vi "Scripting_ChangeNativeBaseClassInSubClass.vi"(0 "SubClass":refnum<vi>, 1 "NewBaseClass":path=path "C:/Projects/Base2_class/Base2.lvclass", 5 "error in (no error)":errorcluster) -> (19 "error out":errorcluster={"status"=TRUE, "code"=1055, "source"="Property Node in Scripting_ConvertBaseClassToSubClass.vi"})   [LabVIEW 2020]
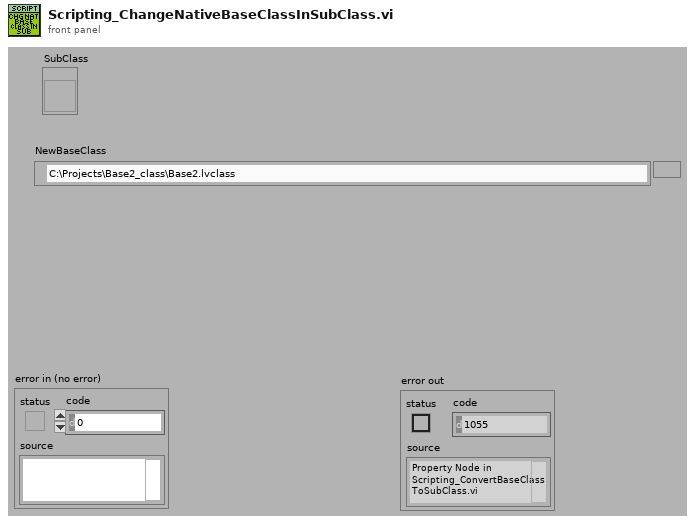
[diagram p1: front panel]
types:
  T1 = cluster{"NewBaseClass":refnum<vi>, "NewBaseClassPath":path, "SubClass":refnum<vi>, "NewBaseClassName":string, "AllBaseClassFiles":path[], "ClassVIs":refnum<vi>[], "CurrentBaseClassRef":refnum<vi>, "CurrentBaseClassPath":path, "CurrentRootBaseClassPath":path, "NewRootBaseClassPath":path, "ProtectedAttrbuts":bool, "ChangeToBase":bool, "App":refnum<vi>}
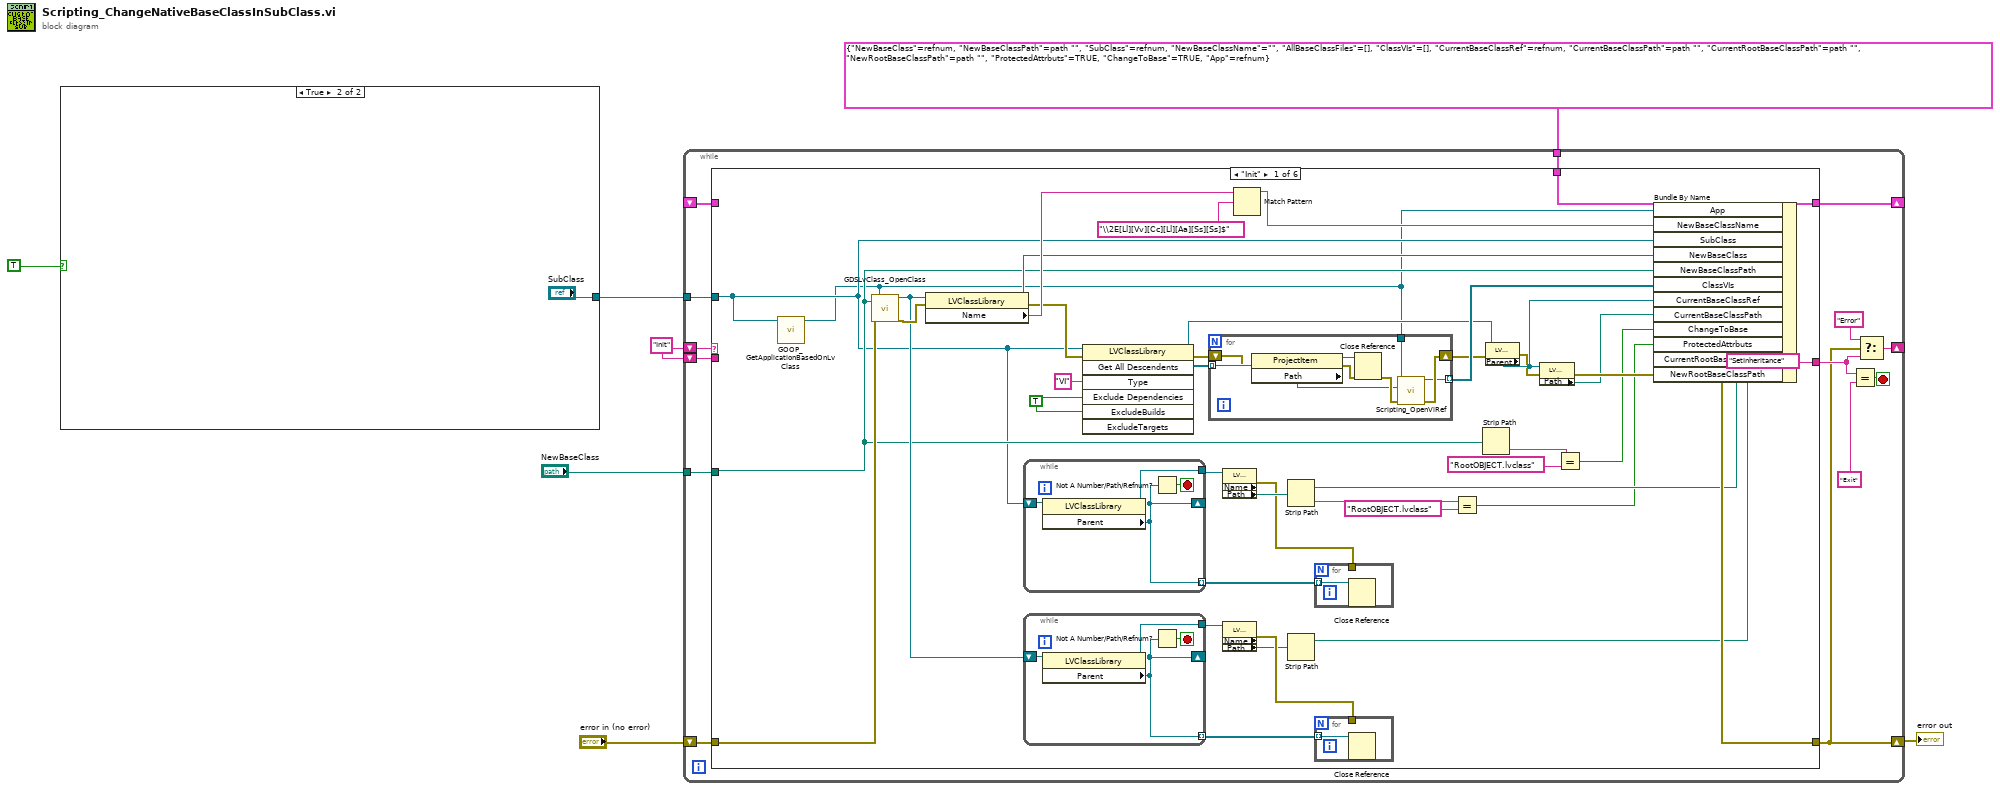
[diagram p0: block diagram]
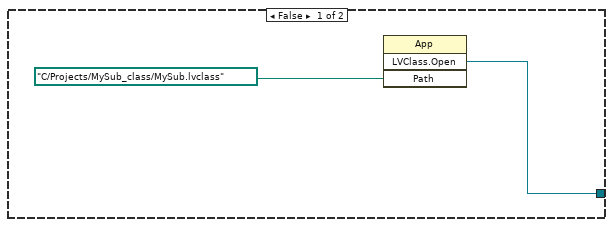
[diagram p2: hidden frame]
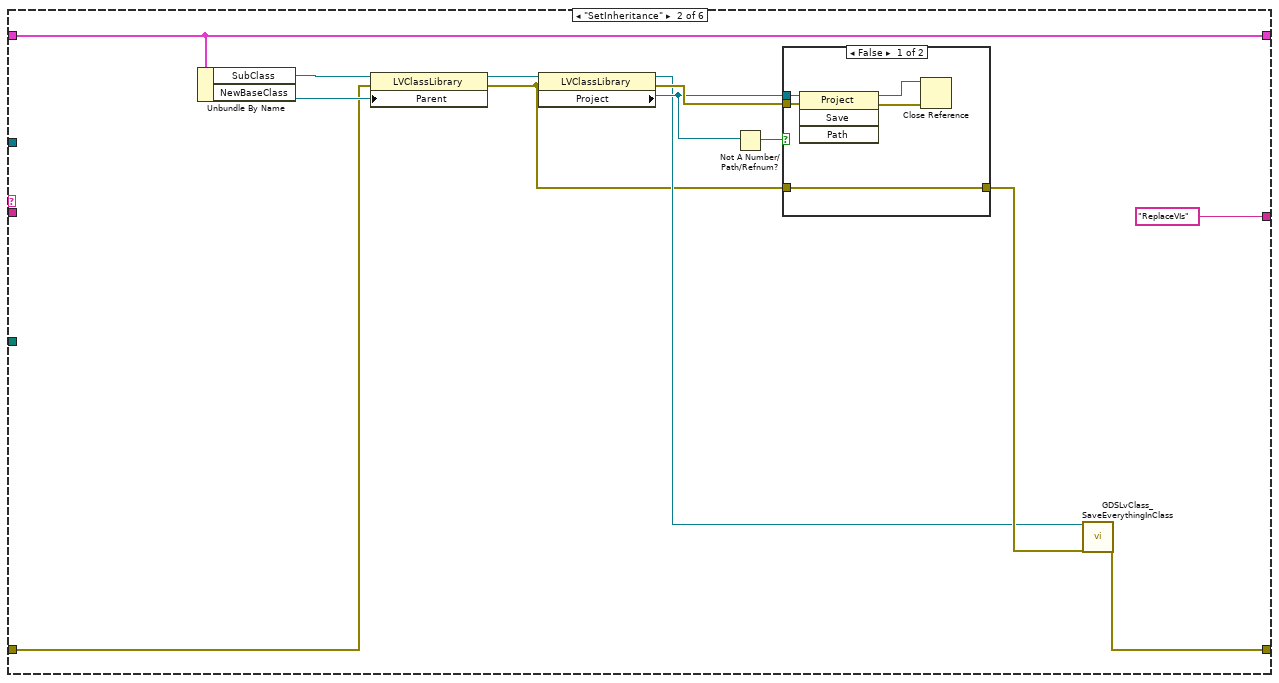
[diagram p3: hidden frame]
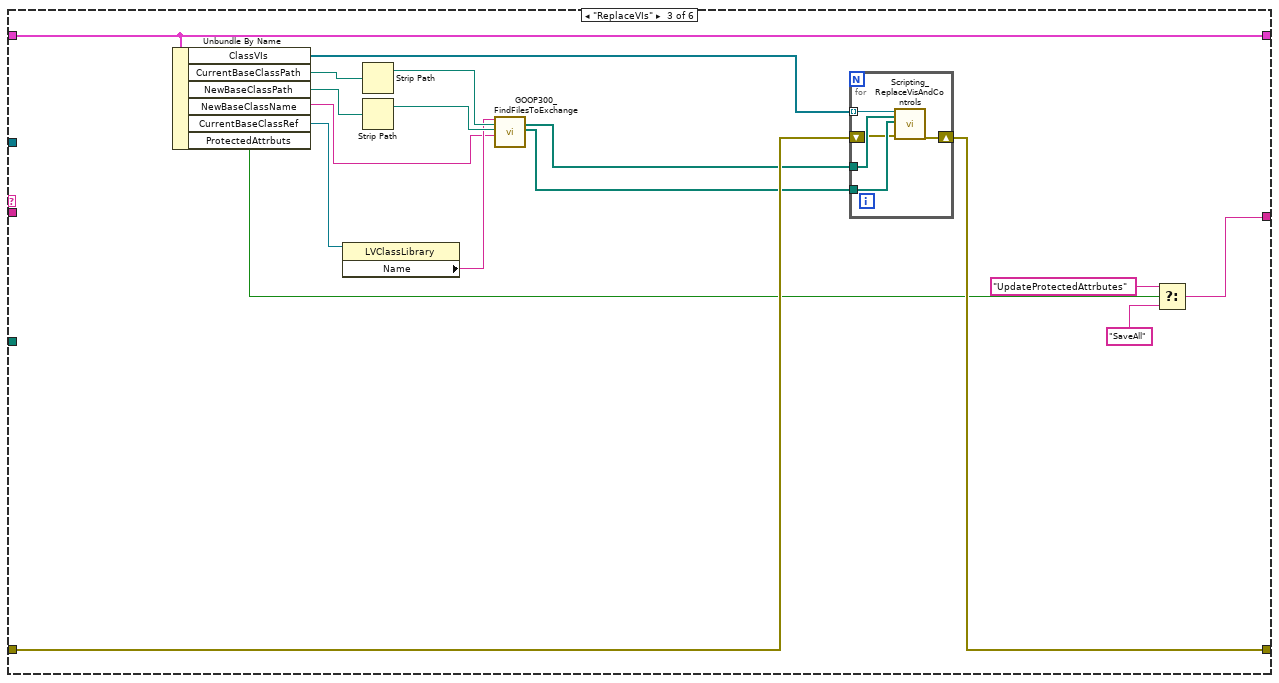
[diagram p5: hidden frame]
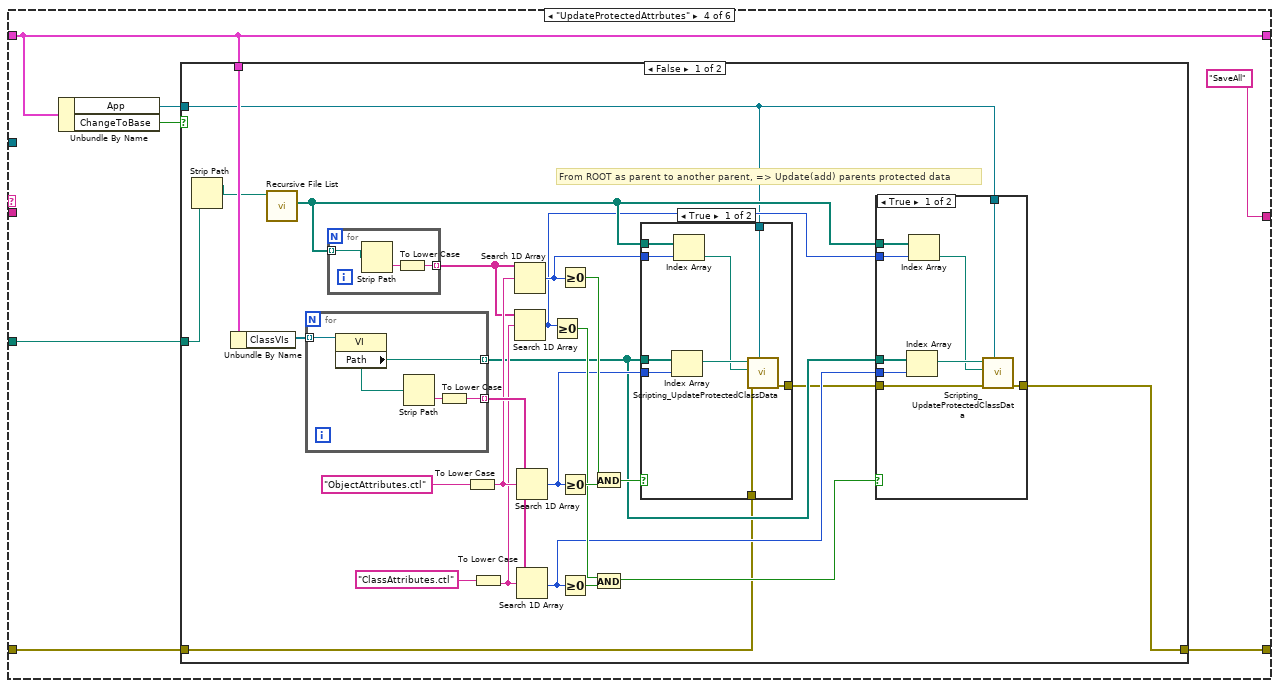
[diagram p6: hidden frame]
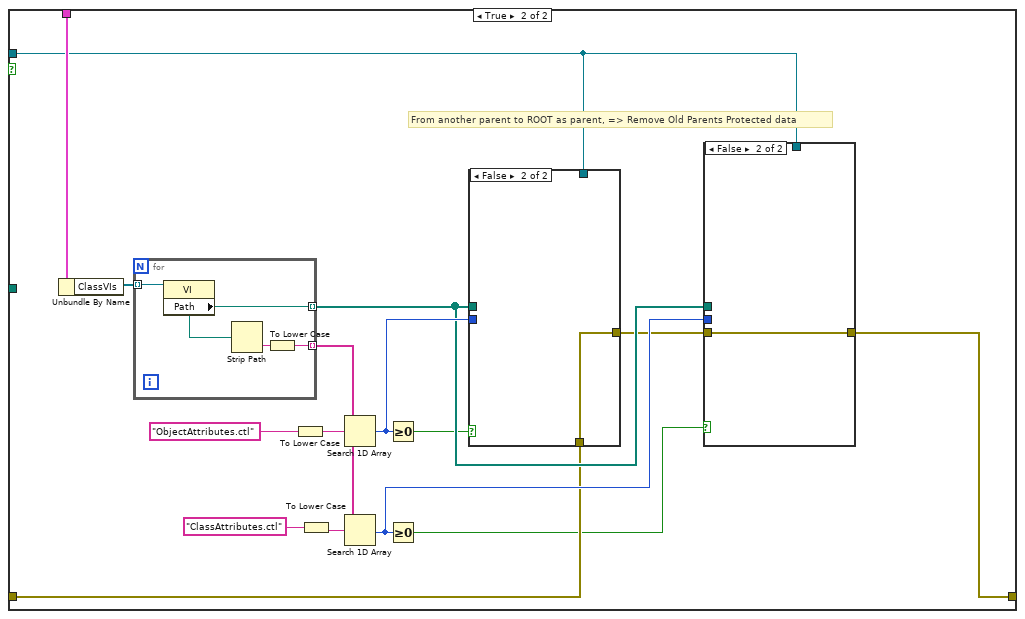
[diagram p9: hidden frame]
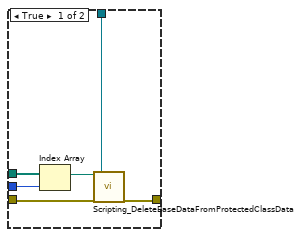
[diagram p10: hidden frame]
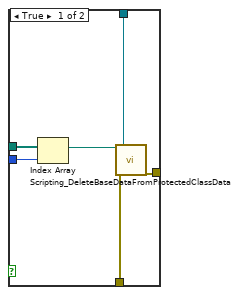
[diagram p11: hidden frame]
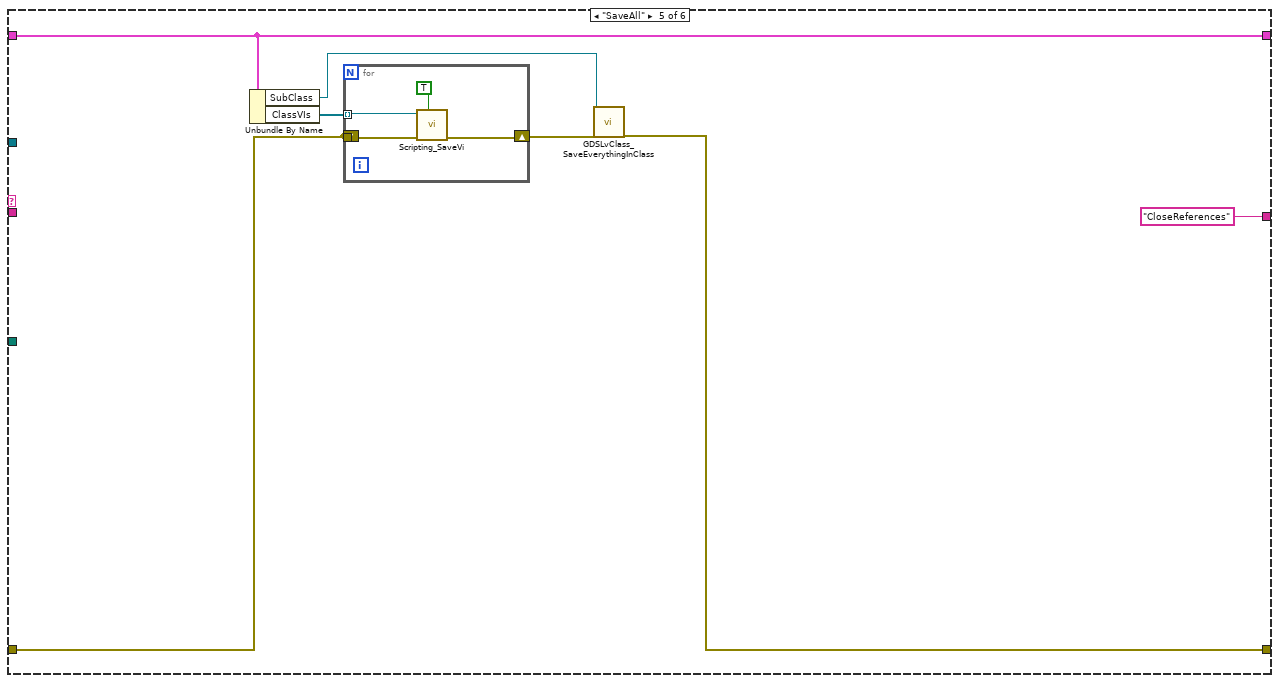
[diagram p12: hidden frame]
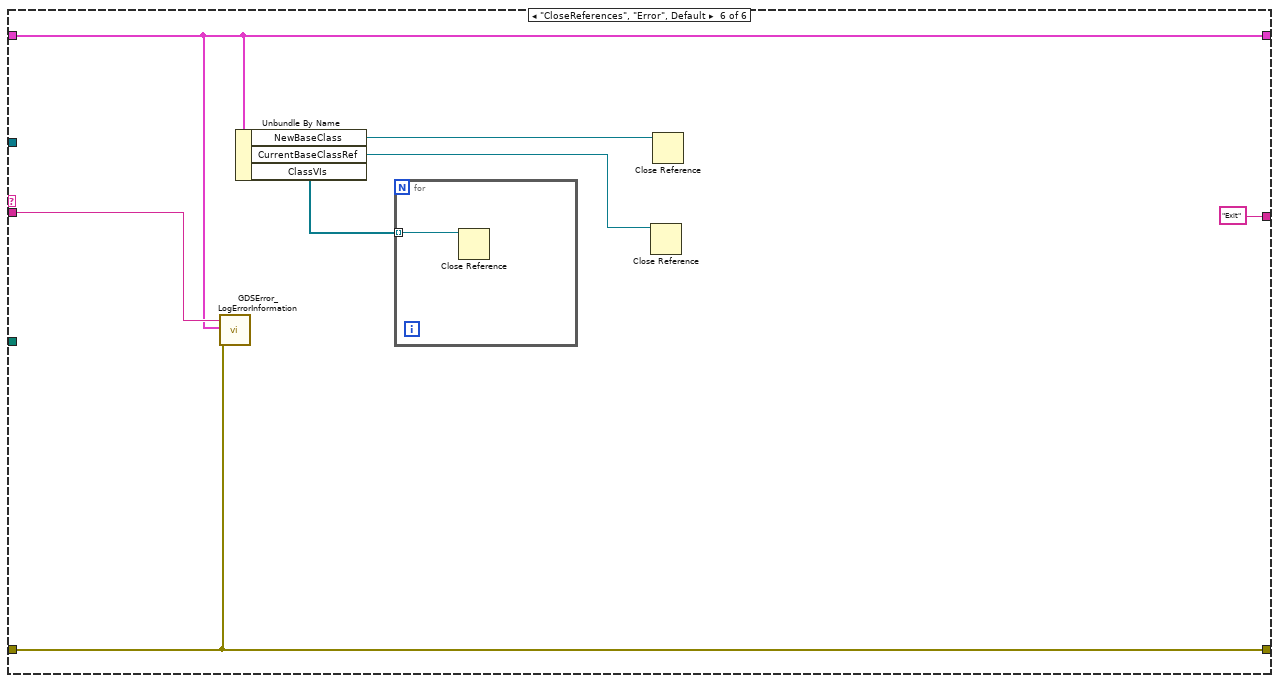
[diagram p13: hidden frame]
diagram:
  w1 = "Init"
  n1 = case shown="True" TRUE {
    tunnel: [w8 "SubClass"] -> w3
    frame False {
      n2 = invoke class="App" method="LVClass.Open"("Path"=path "C:/Projects/MySub_class/MySub.lvclass" ("vi path")) -> ("LVClass.Open"=w8:refnum<vi>)  [unwired: 3 in, 3 out]
    }
    frame True {
    }
  }
  n3 = while {
    shift-right: [w17] -> w6
    shift-left: "error in (no error)" -> [w24]
    shift-right: [w22] -> _
    shift-left: w1 -> [w23]
    shift-right: [w16] -> _
    shift-left: _ -> [w15]
    tunnel: w3 -> [w14]
    tunnel: T1 {"NewBaseClass"=refnum, "NewBaseClassPath"=path "", "SubClass"=refnum, "NewBaseClassName"="", "AllBaseClassFiles"=[], "ClassVIs"=[], "CurrentBaseClassRef"=refnum, "CurrentBaseClassPath"=path "", "CurrentRootBaseClassPath"=path "", "NewRootBaseClassPath"=path "", "ProtectedAttrbuts"=TRUE, "ChangeToBase"=TRUE, "App"=refnum} -> [w13]
    tunnel: "NewBaseClass" -> [w12]
    shift-left: w1 -> [w11]
    stop <- w21 stop-if-true
    n4 = case shown="\"Init\"" w23 {
      tunnel: w24 -> [w48 w94 w114 w132 w224 w233]
      tunnel: [w55 w85 w108 w129 w221 w233] -> w17
      tunnel: ["SetInheritance" "ReplaceVIs" w106 "SaveAll" "CloseReferences" "Exit"] -> w18
      tunnel: [w65 w96 w118 w128 w225 w231] -> w16
      tunnel: w15 -> [_ w96 w118 w128 w225 w231]
      tunnel: w14 -> [w26 _ _ _ _ _]
      tunnel: w13 -> [w62 _ _ _ _ _]
      tunnel: w12 -> [w31 _ _ w131 _ _]
      tunnel: w11 -> [_ _ _ _ _ w232]
      frame "Init" {
        w34 = TRUE ("ExcludeDependencies")
        n5 = call <resource>:"GOOP_GetApplicationBasedOnLvClass.vi"("LVClassLibrary in"=w26) -> ("Application out"=w25:refnum<vi>)  [unwired: 9 in, 1 out]
        n6 = call <resource>:"GDSLvClass_OpenClass.vi"("ClassToOpen"=w31, "error in (no error)"=w48, "Project/ApplicationRef(If empty, currect active project will be used)"=w25) -> ("LVClass.Open"=w36:refnum<vi>, "error out"=w49:errorcluster)  [unwired: 15 in]
        n7 = property class="LVClassLibrary"(reference=w36, error in=w49) -> (reference out=w46:refnum<vi>, error out=w47:errorcluster, "Name"=w60:string)
        n8 = while {
          shift-right: [w73] -> _
          shift-left: w26 -> [w74]
          tunnel: [w73] -> w45 mode=indexing
          tunnel: [w72] -> w44
          stop <- w75 stop-if-true
          n9 = property class="LVClassLibrary"(reference=w74) -> (reference out=w72:refnum<vi>, "Parent"=w73:refnum<vi>)  [unwired: 1 in, 1 out]
          n10 = Not A Number/Path/Refnum?(number/path/refnum=w73) -> (NaN/Path/Refnum?=w75:bool)
        }
        n11 = while {
          shift-right: [w68] -> _
          shift-left: w36 -> [w69]
          tunnel: [w68] -> w37 mode=indexing
          tunnel: [w67] -> w38
          stop <- w70 stop-if-true
          n12 = property class="LVClassLibrary"(reference=w69) -> (reference out=w67:refnum<vi>, "Parent"=w68:refnum<vi>)  [unwired: 1 in, 1 out]
          n13 = Not A Number/Path/Refnum?(number/path/refnum=w68) -> (NaN/Path/Refnum?=w70:bool)
        }
        n14 = invoke class="LVClassLibrary" method="Get All Descendents"(reference=w26, error in=w47, "Type"="VI", "Exclude Dependencies"=w34, "ExcludeBuilds"=w34) -> (reference out=w52:refnum<vi>, error out=w63:errorcluster, "All Descendents"=w64:refnum<vi>[])  [unwired: 2 in, 4 out]
        n15 = for {
          tunnel: w64 -> [w84] mode=indexing
          shift-right: [w79] -> w56
          shift-left: w63 -> [w81]
          tunnel: [w77] -> w57 mode=indexing
          tunnel: w25 -> [w76]
          n16 = property class="ProjectItem"(reference=w84, error in=w81) -> (reference out=w83:refnum<vi>, error out=w82:errorcluster, "Path"=w78:path)
          n17 = Close Reference(reference=w83, error in (no error)=w82) -> (error out=w80:errorcluster)
          n18 = call <resource>:"Scripting_OpenViRef.vi"("error in"=w80, "ViPath/ViName/Viref"=w78, "AppRef"=w76) -> ("error out"=w79:errorcluster, "vi reference"=w77:refnum<vi>)  [unwired: 6 in, 1 out]
        }
        n19 = property class="LVClassLibrary" props=["Name", "Path"](reference=w44) -> (error out=w42:errorcluster, "Path"=w43:path)  [unwired: 1 in, 2 out]
        n20 = property class="LVClassLibrary" props=["Name", "Path"](reference=w38) -> (error out=w40:errorcluster, "Path"=w39:path)  [unwired: 1 in, 2 out]
        n21 = Match Pattern(string=w60, regular expression="\\2E[Ll][Vv][Cc][Ll][Aa][Ss][Ss]$") -> (before substring=w59:string)  [unwired: 1 in, 3 out]
        n22 = Strip Path(path=w43) -> (stripped path=w41:path, name=w33:string)
        n23 = Strip Path(path=w39) -> (stripped path=w35:path)  [unwired: 1 out]
        n24 = for {
          tunnel: w45 -> [w71] mode=indexing
          tunnel: w42 -> [_]
          n25 = Close Reference(reference=w71) -> ()  [unwired: 1 in, 1 out]
        }
        n26 = for {
          tunnel: w37 -> [w66] mode=indexing
          tunnel: w40 -> [_]
          n27 = Close Reference(reference=w66) -> ()  [unwired: 1 in, 1 out]
        }
        n28 = Equal?(x=w33, y="RootOBJECT.lvclass") -> (x = y?=w27:bool)
        n29 = Strip Path(path=w31) -> (name=w30:string)  [unwired: 1 out]
        n30 = property class="LVClassLibrary"(reference=w52, error in=w56) -> (error out=w51:errorcluster, "Parent"=w54:refnum<vi>)  [unwired: 1 out]
        n31 = property class="LVClassLibrary"(reference=w54, error in=w51) -> (error out=w55:errorcluster, "Path"=w53:path)  [unwired: 1 out]
        n32 = Equal?(x=w30, y="RootOBJECT.lvclass") -> (x = y?=w28:bool)
        n33 = Bundle By Name(cluster=w62, "App"=w25, "NewBaseClassName"=w59, "SubClass"=w26, "NewBaseClass"=w46, "NewBaseClassPath"=w31, "ClassVIs"=w57, "CurrentBaseClassRef"=w54, "CurrentBaseClassPath"=w53, "ChangeToBase"=w28, "ProtectedAttrbuts"=w27, "CurrentRootBaseClassPath"=w41, "NewRootBaseClassPath"=w35) -> (w65:T1)
      }
      frame "SetInheritance" {
        n34 = Unbundle By Name(w96) -> ("SubClass"=w97:refnum<vi>, "NewBaseClass"=w95:refnum<vi>)
        n35 = property class="LVClassLibrary"(reference=w97, error in=w94, "Parent"=w95) -> (reference out=w92:refnum<vi>, error out=w86:errorcluster)
        n36 = property class="LVClassLibrary"(reference=w92, error in=w86) -> (reference out=w87:refnum<vi>, error out=w91:errorcluster, "Project"=w90:refnum<vi>)
        n37 = Not A Number/Path/Refnum?(number/path/refnum=w90) -> (NaN/Path/Refnum?=w89:bool)
        n38 = case shown="False" w89 {
          tunnel: w91 -> [w100 _]
          tunnel: w90 -> [w99 _]
          tunnel: w86 -> [w98 w103]
          tunnel: [w98 w103] -> w88
          frame False {
            n39 = invoke class="Project" method="Save"(reference=w99, error in=w100) -> (reference out=w101:refnum<vi>, error out=w102:errorcluster)  [unwired: 2 in, 2 out]
            n40 = Close Reference(reference=w101, error in (no error)=w102) -> ()  [unwired: 1 out]
          }
          frame True {
          }
        }
        n41 = call <resource>:"GDSLvClass_SaveEverythingInClass.vi"("ClassRefIn"=w87, "error in"=w88) -> ("error out"=w85:errorcluster)  [unwired: 16 in, 1 out]
      }
      frame "ReplaceVIs" {
        n42 = Unbundle By Name(w118) -> ("ClassVIs"=w117:refnum<vi>[], "CurrentBaseClassPath"=w120:path, "NewBaseClassPath"=w119:path, "NewBaseClassName"=w109:string, "CurrentBaseClassRef"=w111:refnum<vi>, "ProtectedAttrbuts"=w107:bool)
        n43 = property class="LVClassLibrary"(reference=w111) -> ("Name"=w110:string)  [unwired: 1 in, 2 out]
        n44 = Strip Path(path=w120) -> (stripped path=w116:path)  [unwired: 1 out]
        n45 = Strip Path(path=w119) -> (stripped path=w115:path)  [unwired: 1 out]
        n46 = call <resource>:"GOOP300_FindFilesToExchange.vi"("OldClassName(Prefix or suffix for some VIs)"=w110, "OldFolderPath"=w116, "NewFolderPath"=w115, "NewClassName(Prefix or suffix for some VIs)"=w109) -> ("OldFiles"=w113:path[], "NewFileArray"=w112:path[])  [unwired: 14 in]
        n47 = for {
          shift-right: [w125] -> w108
          shift-left: w114 -> [w122]
          tunnel: w113 -> [w124]
          tunnel: w112 -> [w123]
          tunnel: w117 -> [w121] mode=indexing
          n48 = call <resource>:"Scripting_ReplaceVisAndControls.vi"("ViRef"=w121, "OldVIsAndControls"=w124, "NewVIsAndControls"=w123, "error in (no error)"=w122) -> ("error out"=w125:errorcluster)  [unwired: 14 in, 1 out]
        }
        n49 = Select(t="UpdateProtectedAttrbutes", s=w107, f="SaveAll") -> (s? t:f=w106:string)
      }
      frame "UpdateProtectedAttrbutes" {
        n50 = Unbundle By Name(w128) -> ("App"=w126:refnum<vi>, "ChangeToBase"=w130:bool)
        n51 = case shown="False" w130 {
          tunnel: w132 -> [w138 w191]
          tunnel: w128 -> [w137 w190]
          tunnel: w131 -> [w135 _]
          tunnel: [w134 w189] -> w129
          tunnel: w126 -> [w133 w186]
          frame False {
            # "From ROOT as parent to another parent, => Update(add) parents protected data"
            n52 = Strip Path(path=w135) -> (stripped path=w136:path)  [unwired: 1 out]
            n53 = Unbundle By Name(w137) -> ("ClassVIs"=w158:refnum<vi>[])
            n54 = call <vilib>:"Recursive File List.vi"("Folder Path"=w136) -> ("All Files in Dir"=w144:path[])  [unwired: 6 in, 4 out]
            n55 = for {
              tunnel: w158 -> [w185] mode=indexing
              tunnel: [w184] -> w141 mode=indexing
              tunnel: [w182] -> w156 mode=indexing
              n56 = property class="VI"(reference=w185) -> ("Path"=w184:path)  [unwired: 1 in, 2 out]
              n57 = Strip Path(path=w184) -> (name=w183:string)  [unwired: 1 out]
              n58 = To Lower Case(string=w183) -> (all lower case string=w182:string)
            }
            n59 = for {
              tunnel: w144 -> [w170] mode=indexing
              tunnel: [w169] -> w150 mode=indexing
              n60 = Strip Path(path=w170) -> (name=w171:string)  [unwired: 1 out]
              n61 = To Lower Case(string=w171) -> (all lower case string=w169:string)
            }
            n62 = To Lower Case(string="ObjectAttributes.ctl") -> (all lower case string=w154:string)
            n63 = To Lower Case(string="ClassAttributes.ctl") -> (all lower case string=w149:string)
            n64 = Search 1D Array(1D array=w150, element=w154) -> (index of element=w145:i32)  [unwired: 1 in]
            n65 = Search 1D Array(1D array=w150, element=w149) -> (index of element=w143:i32)  [unwired: 1 in]
            n66 = Search 1D Array(1D array=w156, element=w154) -> (index of element=w146:i32)  [unwired: 1 in]
            n67 = Search 1D Array(1D array=w156, element=w149) -> (index of element=w140:i32)  [unwired: 1 in]
            n68 = Greater Or Equal To 0?(x=w143) -> (x >= 0?=w148:bool)
            n69 = Greater Or Equal To 0?(x=w145) -> (x >= 0?=w152:bool)
            n70 = Greater Or Equal To 0?(x=w146) -> (x >= 0?=w153:bool)
            n71 = Greater Or Equal To 0?(x=w140) -> (x >= 0?=w147:bool)
            n72 = And(x=w152, y=w153) -> (x .and. y?=w151:bool)
            n73 = And(x=w148, y=w147) -> (x .and. y?=w142:bool)
            n74 = case shown="True" w151 {
              tunnel: w138 -> [w180 w181]
              tunnel: w141 -> [w179 _]
              tunnel: w144 -> [w177 _]
              tunnel: w146 -> [w175 _]
              tunnel: w145 -> [w174 _]
              tunnel: [w173 w181] -> w139
              tunnel: w133 -> [w172 _]
              frame True {
                n75 = Index Array(array=w179, index=w175) -> (element=w178:path)
                n76 = Index Array(array=w177, index=w174) -> (element=w176:path)
                n77 = call <resource>:"Scripting_UpdateProtectedClassData.vi"("AppRef"=w172, "error in (no error)"=w180, "NewBaseAttribute"=w176, "BaseAttribute"=w178) -> ("error out"=w173:errorcluster)  [unwired: 6 in, 1 out]
              }
              frame False {
              }
            }
            n78 = case shown="True" w142 {
              tunnel: w141 -> [w167 _]
              tunnel: w144 -> [w165 _]
              tunnel: w140 -> [w163 _]
              tunnel: w143 -> [w162 _]
              tunnel: w139 -> [w161 w168]
              tunnel: [w160 w168] -> w134
              tunnel: w133 -> [w159 _]
              frame True {
                n79 = Index Array(array=w167, index=w163) -> (element=w166:path)
                n80 = Index Array(array=w165, index=w162) -> (element=w164:path)
                n81 = call <resource>:"Scripting_UpdateProtectedClassData.vi"("AppRef"=w159, "error in (no error)"=w161, "NewBaseAttribute"=w164, "BaseAttribute"=w166) -> ("error out"=w160:errorcluster)  [unwired: 6 in, 1 out]
              }
              frame False {
              }
            }
          }
          frame True {
            # "From another parent to ROOT as parent, => Remove Old Parents Protected data"
            n82 = Unbundle By Name(w190) -> ("ClassVIs"=w201:refnum<vi>[])
            n83 = for {
              tunnel: w201 -> [w219] mode=indexing
              tunnel: [w218] -> w194 mode=indexing
              tunnel: [w216] -> w199 mode=indexing
              n84 = property class="VI"(reference=w219) -> ("Path"=w218:path)  [unwired: 1 in, 2 out]
              n85 = Strip Path(path=w218) -> (name=w217:string)  [unwired: 1 out]
              n86 = To Lower Case(string=w217) -> (all lower case string=w216:string)
            }
            n87 = To Lower Case(string="ObjectAttributes.ctl") -> (all lower case string=w197:string)
            n88 = To Lower Case(string="ClassAttributes.ctl") -> (all lower case string=w196:string)
            n89 = Search 1D Array(1D array=w199, element=w197) -> (index of element=w195:i32)  [unwired: 1 in]
            n90 = Search 1D Array(1D array=w199, element=w196) -> (index of element=w193:i32)  [unwired: 1 in]
            n91 = Greater Or Equal To 0?(x=w195) -> (x >= 0?=w187:bool)
            n92 = Greater Or Equal To 0?(x=w193) -> (x >= 0?=w188:bool)
            n93 = case shown="False" w187 {
              tunnel: w191 -> [w211 w215]
              tunnel: w194 -> [w214 _]
              tunnel: w195 -> [w213 _]
              tunnel: [w210 w215] -> w192
              tunnel: w186 -> [w209 _]
              frame True {
                n94 = Index Array(array=w214, index=w213) -> (element=w212:path)
                n95 = call <resource>:"Scripting_DeleteBaseDataFromProtectedClassData.vi"("SubAttribute"=w212, "error in (no error)"=w211, "AppRef"=w209) -> ("error out"=w210:errorcluster)  [unwired: 16 in]
              }
              frame False {
              }
            }
            n96 = case shown="False" w188 {
              tunnel: w194 -> [w207 _]
              tunnel: w193 -> [w206 _]
              tunnel: w192 -> [w204 w208]
              tunnel: [w203 w208] -> w189
              tunnel: w186 -> [w202 _]
              frame True {
                n97 = Index Array(array=w207, index=w206) -> (element=w205:path)
                n98 = call <resource>:"Scripting_DeleteBaseDataFromProtectedClassData.vi"("SubAttribute"=w205, "error in (no error)"=w204, "AppRef"=w202) -> ("error out"=w203:errorcluster)  [unwired: 16 in]
              }
              frame False {
              }
            }
          }
        }
      }
      frame "SaveAll" {
        n99 = Unbundle By Name(w225) -> ("SubClass"=w220:refnum<vi>, "ClassVIs"=w226:refnum<vi>[])
        n100 = for {
          tunnel: w226 -> [w230] mode=indexing
          shift-right: [w227] -> w222
          shift-left: w224 -> [_]
          tunnel: w224 -> [w228]
          n101 = call <resource>:"Scripting_SaveVi.vi"("ForceResaving(False)"=TRUE, "error in (no error)"=w228, "VIRefToSaveIn"=w230) -> ("error out"=w227:errorcluster)  [unwired: 7 in, 1 out]
        }
        n102 = call <resource>:"GDSLvClass_SaveEverythingInClass.vi"("ClassRefIn"=w220, "error in"=w222) -> ("error out"=w221:errorcluster)  [unwired: 16 in, 1 out]
      }
      frame "CloseReferences", "Error", Default {
        n103 = call <resource>:"GDSError_LogErrorInformation.vi"("State"=w232, "LocalVariableData"=w231, "error in (no error)"=w233) -> ()  [unwired: 16 in, 1 out]
        n104 = Unbundle By Name(w231) -> ("NewBaseClass"=w237:refnum<vi>, "CurrentBaseClassRef"=w235:refnum<vi>, "ClassVIs"=w234:refnum<vi>[])
        n105 = for {
          tunnel: w234 -> [w238] mode=indexing
          n106 = Close Reference(reference=w238) -> ()  [unwired: 1 in, 1 out]
        }
        n107 = Close Reference(reference=w235) -> ()  [unwired: 1 in, 1 out]
        n108 = Close Reference(reference=w237) -> ()  [unwired: 1 in, 1 out]
      }
    }
    n109 = Equal?(x=w18, y="Exit") -> (x = y?=w21:bool)
    n110 = Select(t="Error", s=w17, f=w18) -> (s? t:f=w22:string)
  }
  "error out" <- w6
